vi "Get Measure.vi"(8 "error in (no error)":errorcluster caption="entrée d'erreur (pas d'erreur)", 11 "Class LED Analyser in":refnum<class "Class LED Analyser FEASA_3_F.lvclass">) -> (0 "error out":errorcluster caption="sortie d'erreur", 3 "Class LED Analyser Out":refnum<class "Class LED Analyser FEASA_3_F.lvclass">)   [LabVIEW 2020, in "Library Instrument & Equipement.lvlib" / "Library LED Analyser.lvlib" / "Class LED Analyser FEASA_3_F.lvclass"]
uses:
  Class LED Analyser FEASA_3_F.lvclass
  C:/Users/ngarcin/OneDrive - Altyor/Standard TB/Class/Test/Class LED Analyser FEASA/Class LED Analyser FEASA.lvclass
  Class/Test/Class LED Analyser FEASA/Class LED Analyser FEASA.lvclass
  Class LED Analyser FEASA_3_F.lvclass/Class LED Analyser FEASA_3_F.ctl
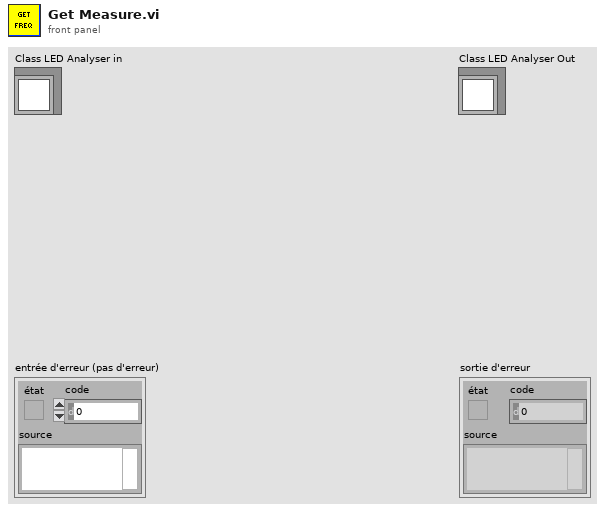
[diagram p1: front panel]
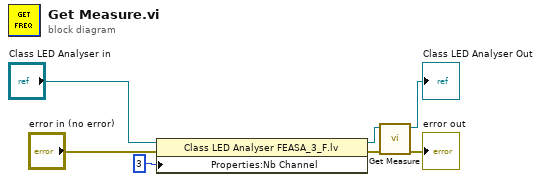
[diagram p0: block diagram]
diagram:
  n1 = property class="Class LED Analyser FEASA_3_F.lv"(reference="Class LED Analyser in", error in="error in (no error)", "Properties:Nb Channel"=u16 3 ("Nb Channel")) -> (reference out=w4:refnum<class "Class LED Analyser FEASA_3_F.lvclass">, error out=w3:errorcluster)
  n2 = call-parent "Get Measure.vi"("error in (no error)"=w3, "Class LED Analyser in"=w4) -> ("error out"=→"error out":errorcluster, "Class LED Analyser Out"=→"Class LED Analyser Out":refnum<class "Class LED Analyser FEASA_3_F.lvclass">)  [unwired: 8 in]
